vi "Build CHM.vi"   [LabVIEW 2018]
uses:
  <vilib>/Utility/config.llb/Read Key (String).vi
  <vilib>/Utility/config.llb/Read Key (Path).vi
  <vilib>/NI/Compiled HTML Menu Tool/CHM Generator/CHM Generator.lvclass
  <vilib>/Utility/config.llb/NI_LVConfig.lvlib
types:
  T1 = typedef "NI_LVConfig.lvlib/Config Data RefNum.ctl" = refnum<k1>
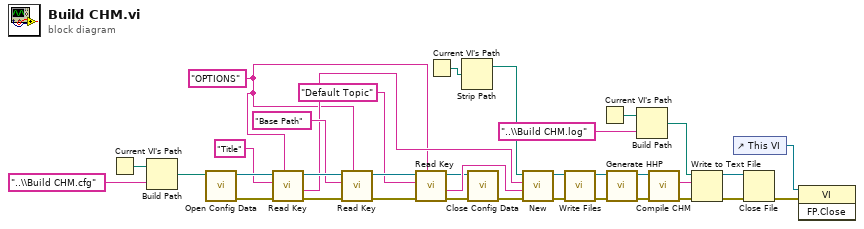
[diagram p0: block diagram]
diagram:
  w16 = "OPTIONS" ("section")
  n1 = Current VI's Path() -> (path=w15:path)
  n2 = Build Path(base path=w15, name or relative path="..\\Build CHM.cfg") -> (appended path=w13:path)
  n3 = call <vilib>:"Open Config Data.vi"("configuration file path"=w13) -> ("error out"=w28:errorcluster, "refnum"=w29:T1)  [unwired: 8 in, 1 out]
  n4 = call-poly <vilib>:"Read Key.vi"("section"=w16, "error in (no error)"=w28, "key"="Title", "refnum"=w29) -> ("error out"=w26:errorcluster, "value"=w23:string, "refnum out"=w25:T1)  [unwired: 4 in, 1 out]
  n5 = call-poly <vilib>:"Read Key.vi"("section"=w16, "error in (no error)"=w26, "key"="Base Path", "refnum"=w25) -> ("error out"=w22:errorcluster, "refnum out"=w21:T1)  [unwired: 4 in, 2 out]
  n6 = call-poly <vilib>:"Read Key.vi"("section"=w16, "error in (no error)"=w22, "key"="Default Topic", "refnum"=w21) -> ("error out"=w18:errorcluster, "value"=w19:string, "refnum out"=w17:T1)  [unwired: 4 in, 1 out]
  n7 = Current VI's Path() -> (path=w2:path)
  n8 = Strip Path(path=w2) -> (stripped path=w1:path)  [unwired: 1 out]
  n9 = call <vilib>:"Close Config Data.vi"("error in (no error)"=w18, "refnum"=w17) -> ("error out"=w3:errorcluster)  [unwired: 8 in, 1 out]
  n10 = call <vilib>:"New.vi"("error in (no error)"=w3, "Default topic"=w19, "Title"=w23, "Base Path"=w1) -> ("error out"=w34:errorcluster, "CHM Generator out"=w35:refnum<class "CHM Generator.lvclass">)  [unwired: 6 in]
  n11 = call-dynamic "Write Files.vi"("error in (no error)"=w34, "CHM Generator in"=w35) -> ("error out"=w33:errorcluster, "CHM Generator out"=w32:refnum<class "CHM Generator.lvclass">)  [unwired: 8 in]
  n12 = Current VI's Path() -> (path=w12:path)
  n13 = call-dynamic "Generate HHP.vi"("error in (no error)"=w33, "CHM Generator in"=w32) -> ("error out"=w30:errorcluster, "CHM Generator out"=w31:refnum<class "CHM Generator.lvclass">)  [unwired: 8 in]
  n14 = Build Path(base path=w12, name or relative path="..\\Build CHM.log") -> (appended path=w10:path)
  n15 = call <vilib>:"Compile CHM.vi"("error in (no error)"=w30, "CHM Generator in"=w31) -> ("error out"=w6:errorcluster, "standard output"=w9:string)  [unwired: 7 in, 1 out]
  n16 = Write to Text File(file (use dialog)=w10, text=w9, error in=w6) -> (refnum out=w7:refnum<file>, error out=w8:errorcluster)  [unwired: 1 in, 1 out]
  n17 = control-ref of="This VI"() -> (w5:refnum<vi>)
  n18 = Close File(refnum=w7, error in=w8) -> (error out=w4:errorcluster)  [unwired: 1 out]
  n19 = invoke class="VI" method="FP.Close"(reference=w5, error in=w4) -> ()  [unwired: 1 in, 3 out]
